vi "RM interrupt timing RT Driver VI.vi"() -> ()   [LabVIEW 2014, in "RM interrupt timing Custom Device.lvlib"]
uses:
  RM interrupt timing Custom Device.lvlib
  <vilib>/NI Veristand/Custom Device API/Custom Device Item Ref.ctl
  Real-Time System Data.ctl
  Configuration Data.ctl
  Channel Data.ctl
  <vilib>/NI Veristand/Custom Device API/Custom Device Channel Type.ctl
  <vilib>/Platform/TimedLoop/XDataNode/timing_clust.ctl
  <vilib>/Platform/TimedLoop/XDataNode/nitl_modes.ctl
  <vilib>/Platform/TimedLoop/XDataNode/wakeup.ctl
  <vilib>/NI Veristand/Custom Device API/Get Item Property (Variant).vi
  <vilib>/platform/TimedLoop/XDataNode/XDataNode.xnode
  <vilib>/NI Veristand/Custom Device API/Custom Device API.lvlib
  <vilib>/NI Veristand/Custom Device Tools/Custom Device Utility Library/Custom Device Utility Library.lvlib
  <vilib>/Platform/TimedLoop/XDataNode/XDNodeRunTimeDep.lvlib
panel:
  in  "Device Clock":string
  in  "Channel Data (DBLs Only)":T1
  in  "Configuration Data":T2
  in  "Real-Time System Data":T3
  in  "Status Notifier":refnum<notifier>
  in  "Device Inputs FIFO":refnum<k33>
  in  "Device Outputs FIFO":refnum<k33>
  in  "Device Reference":T4 format="%.0x"
  # "Custom Device Template\nv1.0"
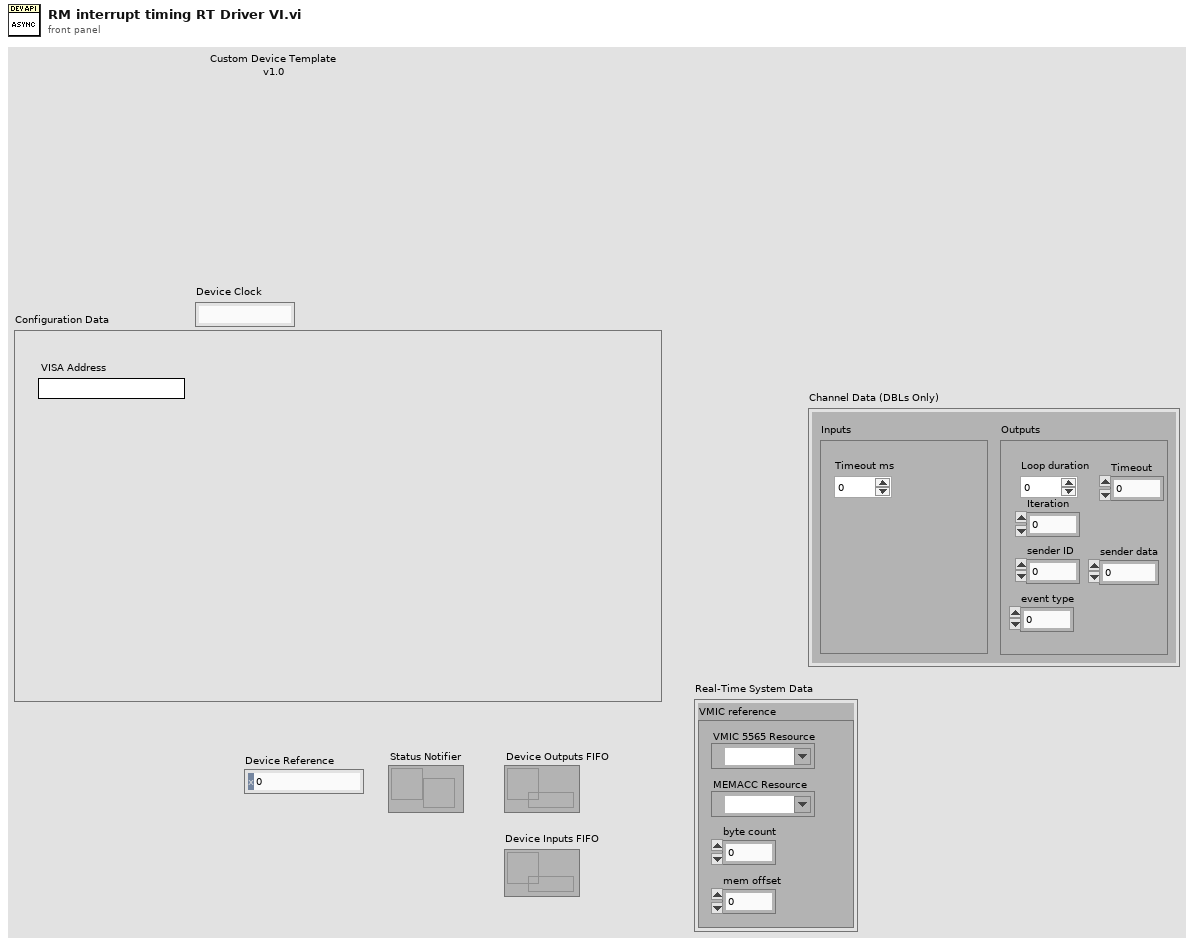
[diagram p1: front panel]
types:
  T1 = typedef "RM interrupt timing Custom Device.lvlib/Channel Data.ctl" = cluster{"Inputs":cluster{"Timeout ms":dbl}, "Outputs":cluster{"Loop duration":dbl, "Iteration":dbl, "Timeout":dbl, "sender data":dbl, "sender ID":dbl, "event type":dbl}}
  T2 = typedef "RM interrupt timing Custom Device.lvlib/Configuration Data.ctl" = cluster{"VISA Address":string}
  T3 = typedef "RM interrupt timing Custom Device.lvlib/Real-Time System Data.ctl" = cluster{"VMIC reference":cluster{"VMIC 5565 Resource":refnum<visa-resource-name>, "MEMACC Resource":refnum<visa-resource-name>, "byte count":u32, "mem offset":u32}}
  T4 = typedef "Custom Device API.lvlib/Custom Device Item Ref.ctl" = u64
  T5 = typedef "Custom Device API.lvlib/Custom Device Channel Type.ctl" = enum16{"Input", "Output"}
  T6 = typedef "XDNodeRunTimeDep.lvlib/timing_clust.ctl" = cluster{"Expected End [f-1]":u64, "Actual End [f-1]":u64, "Finished Late? [f-1]":bool, "Expected End [i-1]":u64, "Actual End [i-1]":u64, "Finished Late? [i-1]":bool, "Expected Start [i]":u64, "Actual Start [i]":u64, "Expected Start [f]":u64, "Actual Start [f]":u64, "Source Name":string, "Structure Name":string, "Period":i64, "Deadline":i64, "Offset":i64, "Start":i64, "Priority":i32, "Timeout":i32, "Mode":T7, "Wakeup Reason":T8, "Error":errorcluster, "Source Type":string, "Secondary Source Type":string, "Global End Time":u64, "Global Start Time":u64, "Frame Duration":u64, "Iteration Duration":u64, "Assigned CPU":i32, "I/O Scan Engine Mode":u32}
  T7 = typedef "XDNodeRunTimeDep.lvlib/nitl_modes.ctl" = enum32{"No Change", "Process missed periods, maintain original phase", "Discard missed periods, maintain original phase", "Process missed periods, ignore original phase", "Discard missed periods, ignore original phase"}
  T8 = typedef "XDNodeRunTimeDep.lvlib/wakeup.ctl" = enum32{"Normal", "Aborted", "Asynchronous wakeup", "Timing source error", "Timed loop error", "Timeout"}
  T9 = cluster{"Loop duration":dbl, "Iteration":dbl, "Timeout":dbl, "sender data":dbl, "sender ID":dbl, "event type":dbl}
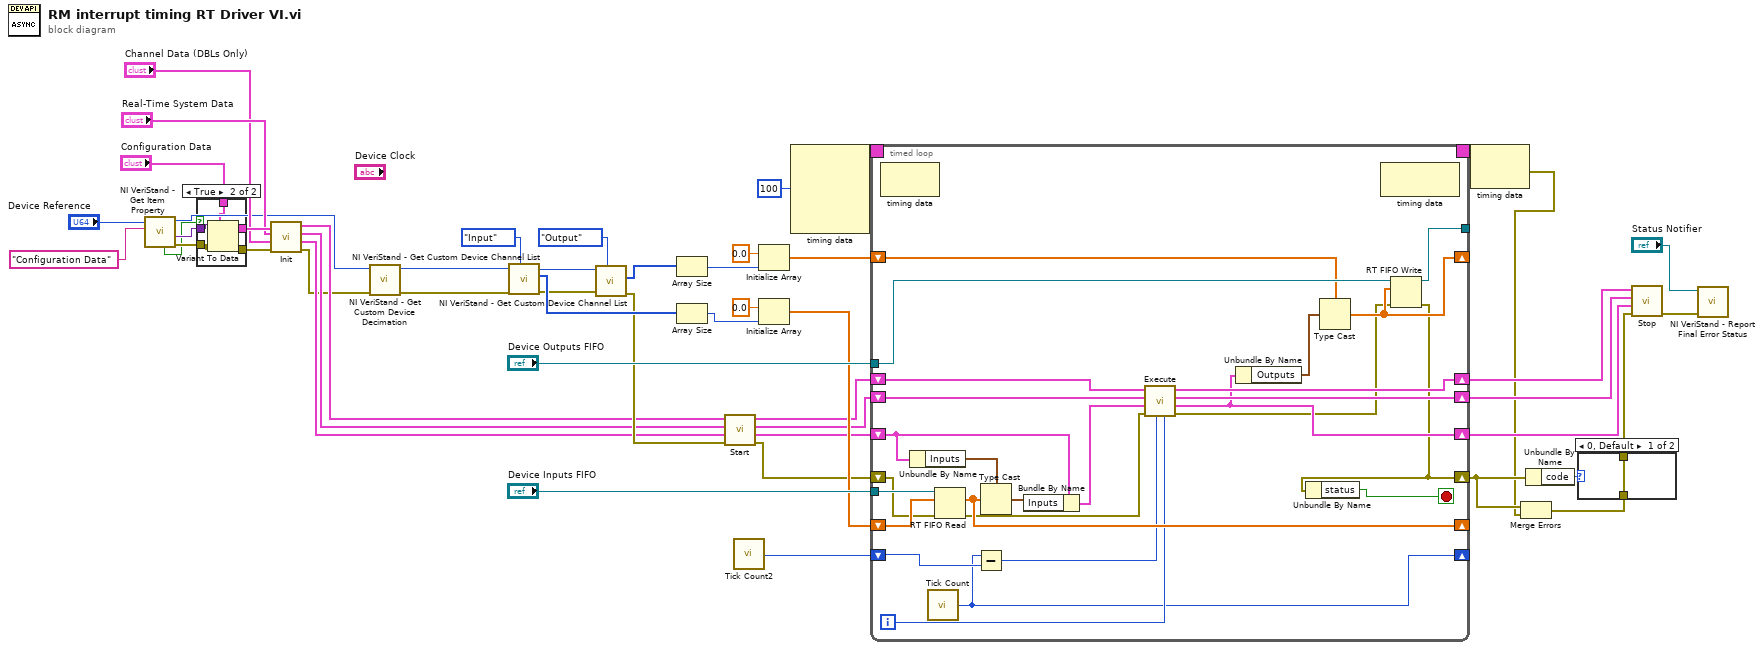
[diagram p0: block diagram]
diagram:
  n1 = call-poly <vilib>:"NI VeriStand - Get Item Property.vi"("Property Name"="Configuration Data", "Item Ref in"="Device Reference") -> ("error out"=w47:errorcluster, "Value"=w46:variant, "Item Ref out"=w17:T4, "Found?"=w12:bool)  [unwired: 6 in]
  n2 = case shown="True" w12 {
    tunnel: w47 -> [w52 w57]
    tunnel: w46 -> [_ w56]
    tunnel: "Configuration Data" -> [w51 w55]
    tunnel: [w51 w54] -> w44
    tunnel: [w52 w53] -> w43
    frame False {
    }
    frame True {
      n3 = Variant To Data(error in=w57, type=w55, Variant=w56) -> (data=w54:T2, error out=w53:errorcluster)
    }
  }
  n4 = call "Init.vi"("error in (no error)"=w43, "Channel Data (DBLs Only)"="Channel Data (DBLs Only)", "Real-Time System Data"="Real-Time System Data", "Configuration Data"=w44) -> ("error out"=w16:errorcluster, "Channel Data (DBLs Only)"=w26:T1, "Real-Time System Data"=w27:T3, "Configuration Data"=w19:T2)  [unwired: 4 in]
  n5 = call <vilib>:"NI VeriStand - Get Custom Device Decimation.vi"("error in (no error)"=w16, "Device Ref in"=w17) -> ("error out"=w14:errorcluster, "Device Ref out"=w15:T4)  [unwired: 7 in, 1 out]
  n6 = call <vilib>:"NI VeriStand - Get Custom Device Channel List.vi"("Channel Type"=Custom_Device_Channel_Type."Input", "error in (no error)"=w14, "Device Ref in"=w15) -> ("error out"=w29:errorcluster, "Specified Channel Ref List"=w39:T4[], "Device Ref out"=w41:T4)  [unwired: 6 in]
  n7 = call <vilib>:"NI VeriStand - Get Custom Device Channel List.vi"("Channel Type"=Custom_Device_Channel_Type."Output", "error in (no error)"=w29, "Device Ref in"=w41) -> ("error out"=w28:errorcluster, "Specified Channel Ref List"=w38:T4[])  [unwired: 6 in, 1 out]
  n8 = Array Size(array=w38) -> (size(s)=w36:i32)
  n9 = Array Size(array=w39) -> (size(s)=w37:i32)
  n10 = call "Start.vi"("error in (no error)"=w28, "Channel Data (DBLs Only)"=w26, "Real-Time System Data"=w27, "Configuration Data"=w19) -> ("error out"=w13:errorcluster, "Channel Data (DBLs Only)"=w25:T1, "Real-Time System Data"=w18:T3, "Configuration Data"=w21:T2)  [unwired: 4 in]
  n11 = call "Tick Count2"() -> ("Tick Count(uSec)"=w6:u32)
  n12 = Initialize Array(0.0 ("element"), w36) -> (w33:dbl[])
  n13 = Initialize Array(0.0 ("element"), w37) -> (w32:dbl[])
  n14 = node-c288(i64 100 ("Period")) -> (w5:T6)  [unwired: 3 in]
  n15 = timed-loop {
    tunnel: "Device Inputs FIFO" -> [w83]
    tunnel: "Device Outputs FIFO" -> [w82]
    tunnel: [w81] -> _
    shift-right: [w73] -> _
    shift-left: w33 -> [w74]
    shift-right: [w72] -> _
    shift-left: w32 -> [w79]
    shift-right: [w70] -> w24
    shift-left: w18 -> [w67]
    shift-right: [w69] -> w23
    shift-left: w25 -> [w78]
    shift-right: [w71] -> w20
    shift-left: w21 -> [w68]
    shift-right: [w62] -> w8
    shift-left: w13 -> [w65]
    shift-right: [w58] -> _
    shift-left: w6 -> [w61]
    timing: w5 -> [_]
    timing-out: [_] -> w4
    i -> [w60]
    stop <- w80 stop-if-true
    n16 = node-c288() -> ()  [unwired: 1 in, 1 out]
    n17 = Unbundle By Name(w78) -> ("Inputs"=w77:cluster{"Timeout ms":dbl})
    n18 = call "Tick Count"() -> ("Tick Count(uSec)"=w58:u32)
    n19 = RT FIFO Read(0:w83, 1:w79, 3:w65) -> (9:w72:dbl[], 11:w64:errorcluster)  [unwired: 1 in, 3 out]
    n20 = Subtract(x=w58, y=w61) -> (x-y=w59:u32)
    n21 = Type Cast(type=w77, x=w72) -> (*(type *) &x=w76:cluster{"Timeout ms":dbl})
    n22 = Bundle By Name(cluster=w78, "Inputs"=w76) -> (w66:T1)
    n23 = call "Execute.vi"("Iteration"=w60, "Time"=w59, "error in (no error)"=w64, "Channel Data (DBLs Only)"=w66, "Real-Time System Data"=w67, "Configuration Data"=w68) -> ("error out"=w63:errorcluster, "Channel Data (DBLs Only)"=w69:T1, "Real-Time System Data"=w70:T3, "Configuration Data"=w71:T2)  [unwired: 2 in]
    n24 = Unbundle By Name(w69) -> ("Outputs"=w75:T9)
    n25 = Type Cast(type=w74, x=w75) -> (*(type *) &x=w73:dbl[])
    n26 = node-c288() -> ()  [unwired: 1 in, 1 out]
    n27 = RT FIFO Write(0:w82, 1:w73, 3:w63) -> (8:w81:refnum<k33>, 11:w62:errorcluster)  [unwired: 2 in, 2 out]
    n28 = Unbundle By Name(w62) -> ("status"=w80:bool)
  }
  n29 = node-c288(w4) -> (w1:errorcluster)
  n30 = Merge Errors(w8, w1) -> (w2:errorcluster)
  n31 = Unbundle By Name(w8) -> ("code"=w9:i32)
  n32 = case shown="0, Default" w9 {
    tunnel: w2 -> [w86 _]
    tunnel: [w86 _] -> w7
    frame 0, Default {
    }
    frame -2206 {
    }
  }
  n33 = call "Stop.vi"("error in (no error)"=w7, "Channel Data (DBLs Only)"=w23, "Real-Time System Data"=w24, "Configuration Data"=w20) -> ("error out"=w11:errorcluster)  [unwired: 7 in]
  n34 = call <vilib>:"NI VeriStand - Report Final Error Status.vi"("error in (no error)"=w11, "Status Notifier"="Status Notifier") -> ()  [unwired: 1 in, 9 out]
